vi "Set ListViewItem SubItems.vi"(8 "error in (no error)":errorcluster caption="错误输入（无错误）", 9 "SubItems":string[](array[string]), 10 "index":i32, 11 "ListViewClass 输入":refnum<class "ListViewClass.lvclass"> caption="DNL_LabVIEW Object in") -> (0 "error out":errorcluster caption="错误输出", 3 "ListViewClass 输出":refnum<class "ListViewClass.lvclass"> caption="DNL_LabVIEW Object out")   [LabVIEW 2012, in "ListViewClass.lvclass"]
uses:
  ListViewClass.lvclass
  System.Windows.Forms
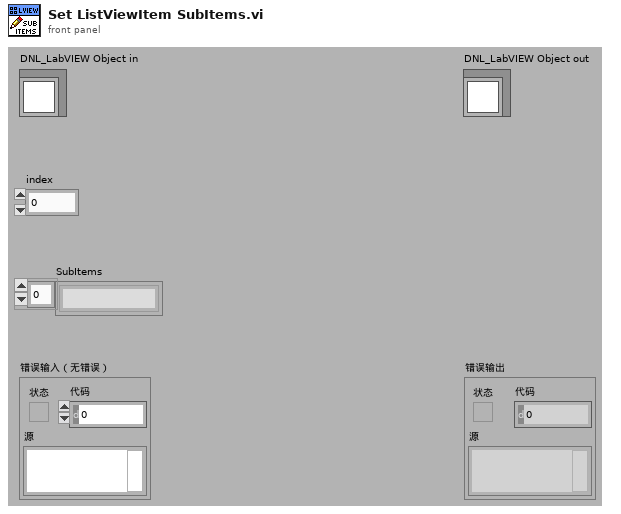
[diagram p1: front panel]
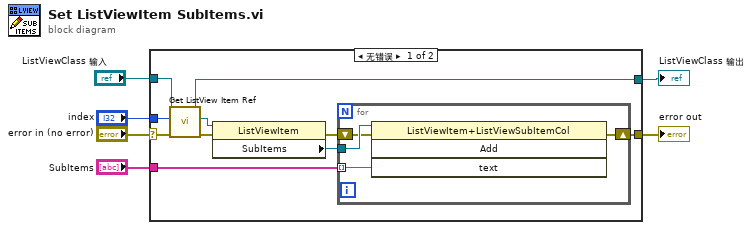
[diagram p0: block diagram]
diagram:
  n1 = case shown="无错误" "error in (no error)" {
    selector: "error in (no error)" -> [w10 w22]
    tunnel: [w13 w22] -> w5
    tunnel: [w8 w21] -> w3
    tunnel: "ListViewClass 输入" -> [w12 w21]
    tunnel: "SubItems" -> [w15 _]
    tunnel: "index" -> [w11 _]
    frame No Error {
      n2 = call "Get ListView Item Ref.vi"("error in (no error)"=w10, "index"=w11, "ListViewClass 输入"=w12) -> ("error out"=w7:errorcluster, "get_Item"=w9:refnum<k24>, "ListViewClass 输出"=w8:refnum<class "ListViewClass.lvclass">)  [unwired: 6 in]
      n3 = property class="ListViewItem"(reference=w9, error in=w7) -> (error out=w14:errorcluster, "SubItems"=w16:refnum<k24>)  [unwired: 1 out]
      n4 = for {
        tunnel: w16 -> [w20]
        tunnel: w15 -> [w19] mode=indexing
        shift-right: [w17] -> w13
        shift-left: w14 -> [w18]
        n5 = invoke class="ListViewItem+ListViewSubItemCol" method="Add"(reference=w20, error in=w18, "text"=w19) -> (error out=w17:errorcluster)  [unwired: 1 in, 3 out]
      }
    }
    frame Error {
    }
  }
  "error out" <- w5
  "ListViewClass 输出" <- w3
